vi "Configure Edge Counter.vi"(8 "error in":errorcluster, 10 "Mode":T1=enum."RISING", 11 "VISA resource name":refnum<visa-resource-name>) -> (0 "error out":errorcluster, 3 "VISA resource name out":refnum<visa-resource-name>)   [LabVIEW 2020, in "BDAQ-6104.lvlib"]
doc: "Configure the counter function on digital input pin 1."
uses:
  <instrlib>/BDAQ-6104/BDAQ-6104.lvlib
  <instrlib>/BDAQ-6104/Private/Edge Triger Type.ctl
panel:
  out "concatenated string":string
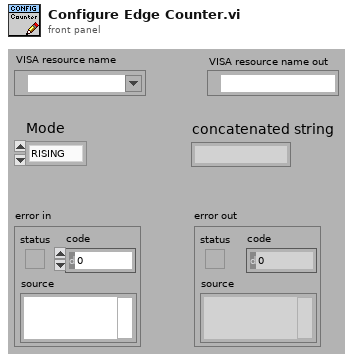
[diagram p1: front panel]
types:
  T1 = typedef "BDAQ-6104.lvlib/Edge Triger Type.ctl" = enum16{"FALLING", "RISING", "CHANGE"}
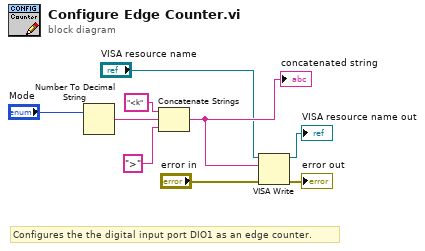
[diagram p0: block diagram]
diagram:
  # "Configures the the digital input port DIO1 as an edge counter."
  n1 = Number To Decimal String(number="Mode") -> (decimal integer string=w8:string)  [unwired: 1 in]
  n2 = Concatenate Strings("<k", w8, ">") -> (w7:string)
  "concatenated string" <- w7
  n3 = VISA Write(VISA resource name="VISA resource name", write buffer=w7, error in (no error)="error in") -> (VISA resource name out=→"VISA resource name out":refnum<visa-resource-name>, error out=→"error out":errorcluster)  [unwired: 1 out]
